vi "GlobalButtons.vi"() -> ()   [LabVIEW 2015]
panel:
  out "ThirdSpeed":bool
  in  "FlipAxis":bool
  in  "Get Image":bool
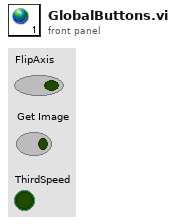
[diagram p1: front panel]
diagram:
